vi "Example.vi"() -> ()   [LabVIEW 2019]
uses:
  Classes/BlueJSONTextSerializer/BlueJSONTextSerializer.lvclass
  <userlib>/Blue Origin/BlueSerialization/BlueSerializer/BlueSerializer.lvclass
  <userlib>/Blue Origin/BlueSerialization/BlueSerializable/BlueSerializable.lvclass
  683d9f73-8691-46f1-ba30-177d53131fe4.vi
  C:/Program Files (x86)/National Instruments/LabVIEW 2019/user.lib/Blue Origin/BlueSerialization/BlueSerializer/BlueSerializer.lvclass
panel:
  out "Data out 2":T1
  out "always true":bool
  out "Serialized Data 2":string
  out "error out 2":errorcluster
  out "Serialized Data 1":string
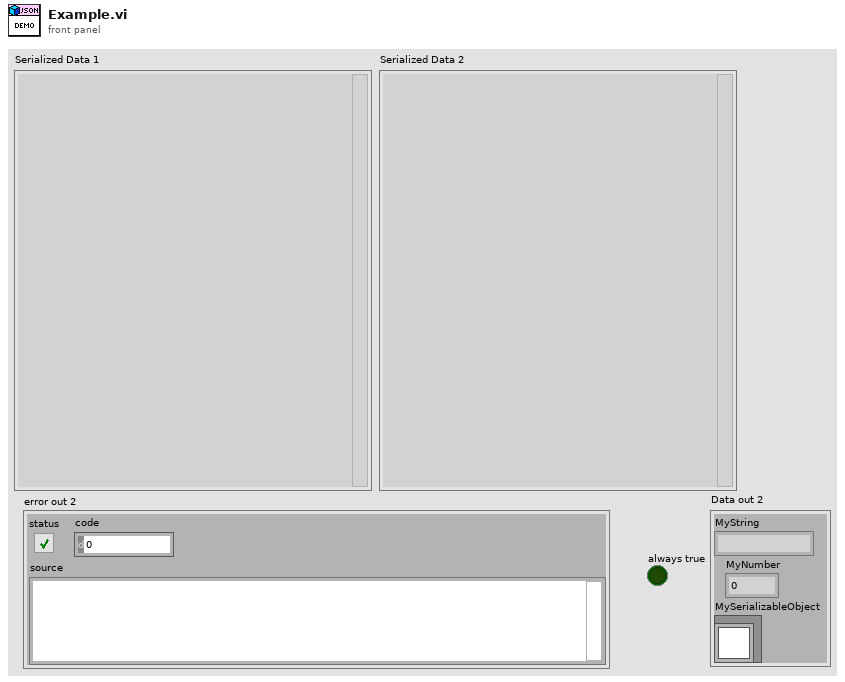
[diagram p1: front panel]
types:
  T1 = cluster{"MyString":string, "MyNumber":dbl, "MySerializableObject":refnum<class "BlueSerializable.lvclass">}
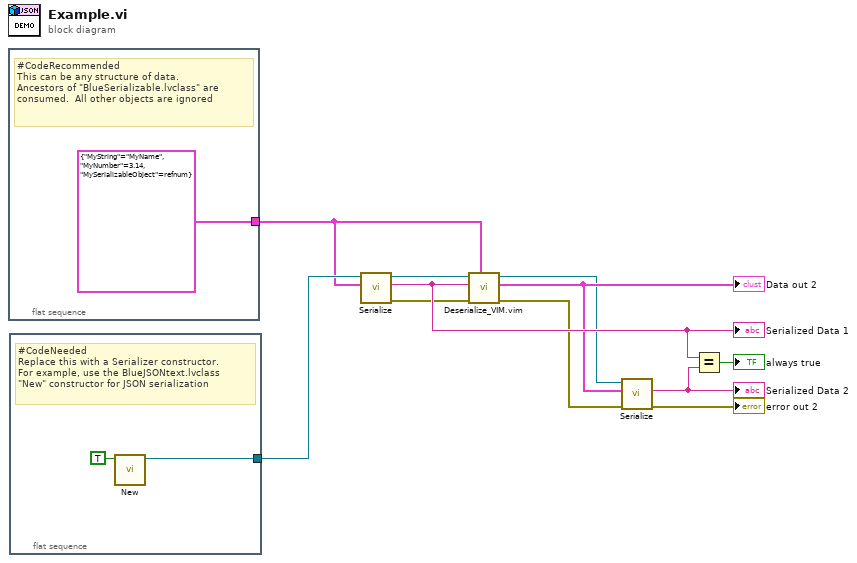
[diagram p0: block diagram]
diagram:
  n1 = flat-sequence {
    tunnel: [T1 {"MyString"="MyName", "MyNumber"=3.14, "MySerializableObject"=refnum}] -> w4
    frame #0 {
      # "#CodeRecommended\nThis can be any structure of data.\nAncestors of \"BlueSerializable.lvclass\" are consumed.  All other objects are ignored"
    }
  }
  n2 = flat-sequence {
    tunnel: [w13] -> w8
    frame #0 {
      # "#CodeNeeded\nReplace this with a Serializer constructor.\nFor example, use the BlueJSONtext.lvclass\n\"New\" constructor for JSON serialization"
      n3 = call "New.vi"("PrettyPrint?"=TRUE) -> ("BlueJSONTextSerializer out"=w13:refnum<class "BlueJSONTextSerializer.lvclass">)  [unwired: 9 in, 1 out]
    }
  }
  n4 = call <userlib>:"Serialize.vi"("Anything"=w4, "BlueSerializer in"=w8) -> ("error out"=w5:errorcluster, "Serialized Text"=w6:string, "BlueSerializer out"=w7:refnum<class "BlueJSONTextSerializer.lvclass">)  [unwired: 7 in]
  "Serialized Data 1" <- w6
  n5 = call "Deserialize_VIM.vim"("Anything"=w4, "error in (no error)"=w5, "Serialized Text"=w6, "BlueSerializer in"=w7) -> ("error out"=w3:errorcluster, "Data out"=w2:T1, "BlueSerializer out"=w1:refnum<class "BlueJSONTextSerializer.lvclass">)  [unwired: 5 in]
  "Data out 2" <- w2
  n6 = call <userlib>:"Serialize.vi"("error in (no error)"=w3, "Anything"=w2, "BlueSerializer in"=w1) -> ("error out"=→"error out 2":errorcluster, "Serialized Text"=w10:string)  [unwired: 6 in, 1 out]
  "Serialized Data 2" <- w10
  n7 = Equal?(x=w6, y=w10) -> (x = y?=→"always true":bool)
